vi "PID.vi"(6 "reinitialize? (F)":bool, 7 "output range":cluster{"output high":dbl, "output low":dbl}={"output high"=100.0, "output low"=-100.0} {"output low" format="%.2f"; "output high" format="%.2f"}, 8 "dt (s)":dbl=-1.0 format="%.3f", 9 "PID gains":T1={"proportional gain (Kc)"=1.0, "integral time (Ti, min)"=0.01, "derivative time (Td, min)"=0.0} {"derivative time (Td, min)" format="%.3f"; "integral time (Ti, min)" format="%.3f"; "proportional gain (Kc)" format="%.3f"}, 10 "process variable":dbl format="%.2f", 11 "setpoint":dbl format="%.2f") -> (2 "output":dbl format="%.2f")   [LabVIEW 2012]
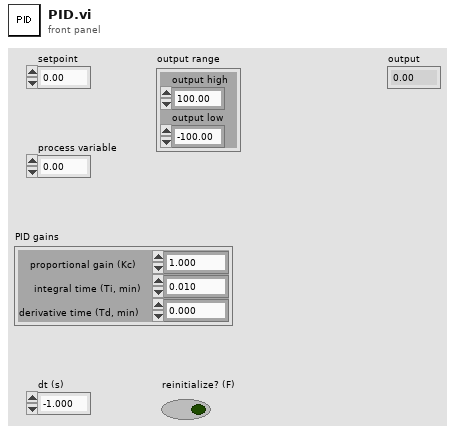
[diagram p1: front panel]
types:
  T1 = cluster{"proportional gain (Kc)":dbl, "integral time (Ti, min)":dbl, "derivative time (Td, min)":dbl}
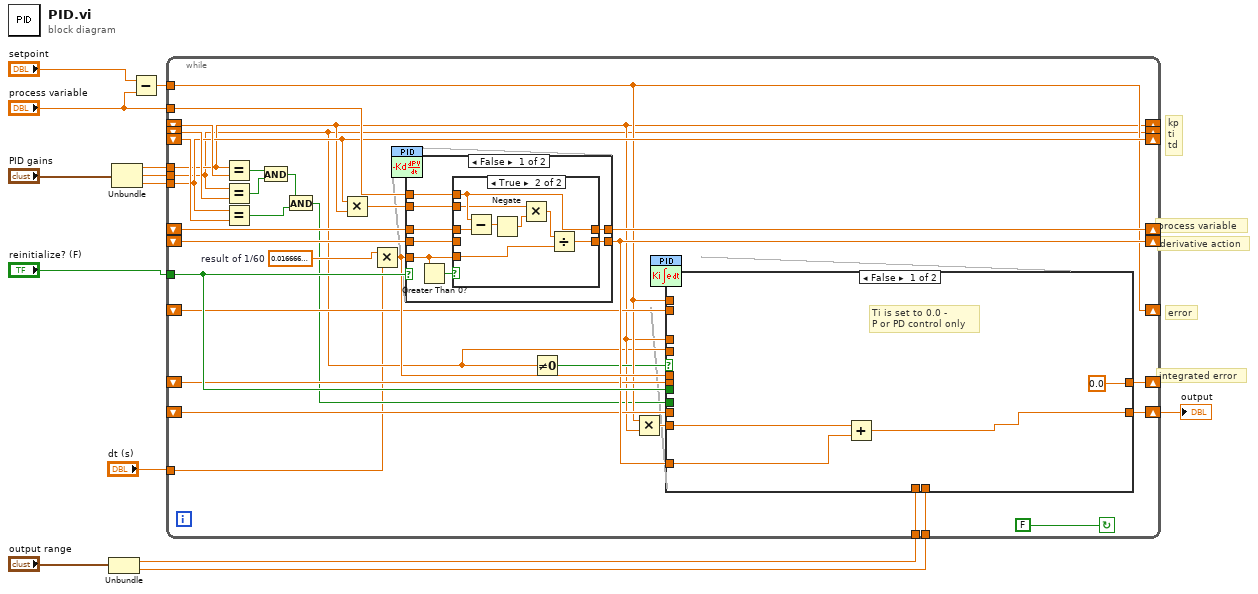
[diagram p0: block diagram]
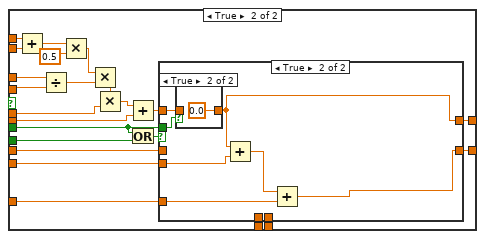
[diagram p2: hidden frame]
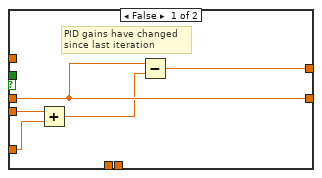
[diagram p3: hidden frame]
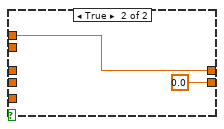
[diagram p6: hidden frame]
diagram:
  # "derivative action"
  # "process variable"
  # "kp\nti\ntd"
  # "error"
  # "integrated error"
  n1 = Unbundle("output range") -> ("output high"=w10:dbl, "output low"=w9:dbl)
  n2 = Unbundle("PID gains") -> ("proportional gain (Kc)"=w13:dbl, "integral time (Ti, min)"=w12:dbl, "derivative time (Td, min)"=w11:dbl)
  n3 = Subtract(x="setpoint", y="process variable") -> (x-y=w2:dbl)
  n4 = while {
    tunnel: "reinitialize? (F)" -> [w45]
    shift-right: [w21] -> _
    shift-left: _ -> [w27]
    shift-right: [w20] -> _
    shift-left: _ -> [w42]
    shift-right: [w25] -> _
    shift-left: _ -> [w43]
    tunnel: w13 -> [w21]
    tunnel: w12 -> [w20]
    tunnel: w11 -> [w25]
    tunnel: "dt (s)" -> [w14]
    tunnel: w10 -> [w41]
    tunnel: w9 -> [w40]
    tunnel: "process variable" -> [w39]
    shift-right: [w38] -> _
    shift-left: _ -> [w37]
    shift-right: [w36] -> _
    shift-left: _ -> [w30]
    shift-right: [w35] -> w6
    shift-left: _ -> [w34]
    shift-right: [w24] -> _
    shift-left: _ -> [w33]
    shift-right: [w32] -> _
    shift-left: _ -> [w31]
    tunnel: w2 -> [w24]
    stop <- FALSE continue-if-true
    w23 = 0.016666666666666666  # result of 1/60
    n5 = Equal?(x=w21, y=w27) -> (x = y?=w19:bool)
    n6 = Equal?(x=w20, y=w42) -> (x = y?=w18:bool)
    n7 = Equal?(x=w25, y=w43) -> (x = y?=w16:bool)
    n8 = And(x=w19, y=w18) -> (x .and. y?=w17:bool)
    n9 = And(x=w17, y=w16) -> (x .and. y?=w15:bool)
    n10 = Multiply(x=w25, y=w21) -> (x*y=w29:dbl)
    n11 = Multiply(x=w23, y=w14) -> (x*y=w44:dbl)
    n12 = case shown="False" w45 {
      tunnel: w37 -> [w94 _]
      tunnel: w29 -> [w91 _]
      tunnel: w39 -> [w93 w106]
      tunnel: [w90 w106] -> w38
      tunnel: [w92 0.0] -> w36
      tunnel: w30 -> [w88 _]
      tunnel: w44 -> [w87 _]
      frame False {
        n13 = Greater Than 0?(x=w87) -> (x > 0?=w89:bool)
        n14 = case shown="True" w89 {
          tunnel: w94 -> [w96 w102]
          tunnel: w87 -> [_ w101]
          tunnel: w93 -> [_ w99]
          tunnel: [w95 w100] -> w92
          tunnel: w91 -> [_ w97]
          tunnel: [w96 w99] -> w90
          tunnel: w88 -> [w95 _]
          frame False {
            # "dt = 0 min"
          }
          frame True {
            n15 = Subtract(x=w99, y=w102) -> (x-y=w104:dbl)
            n16 = Negate(x=w104) -> (-x=w98:dbl)
            n17 = Multiply(x=w97, y=w98) -> (x*y=w103:dbl)
            n18 = Divide(x=w103, y=w101) -> (x/y=w100:dbl)
          }
        }
      }
      frame True {
      }
    }
    n19 = Not Equal To 0?(x=w20) -> (x != 0?=w22:bool)
    n20 = Multiply(x=w24, y=w21) -> (x*y=w28:dbl)
    n21 = case shown="False" w22 {
      tunnel: w24 -> [_ w71]
      tunnel: w33 -> [_ w72]
      tunnel: w31 -> [_ w69]
      tunnel: [0.0 w64] -> w32
      tunnel: w28 -> [w49 w67]
      tunnel: [w46 w63] -> w35
      tunnel: w34 -> [_ w65]
      tunnel: w36 -> [w48 w62]
      tunnel: w45 -> [_ w61]
      tunnel: w15 -> [_ w60]
      tunnel: w44 -> [_ w52]
      tunnel: w41 -> [_ w58]
      tunnel: w40 -> [_ w59]
      tunnel: w21 -> [_ w56]
      tunnel: w20 -> [_ w55]
      frame False {
        # "Ti is set to 0.0 -\nP or PD control only"
        n22 = Add(x=w49, y=w48) -> (x+y=w46:dbl)
      }
      frame True {
        n23 = Add(x=w71, y=w72) -> (x+y=w70:dbl)
        n24 = Divide(x=w56, y=w55) -> (x/y=w53:dbl)
        n25 = Multiply(x=w70, y=0.5) -> (x*y=w54:dbl)
        n26 = Multiply(x=w54, y=w53) -> (x*y=w51:dbl)
        n27 = Multiply(x=w51, y=w52) -> (x*y=w50:dbl)
        n28 = Add(x=w50, y=w69) -> (x+y=w68:dbl)
        n29 = Or(x=w61, y=w60) -> (x .or. y?=w66:bool)
        n30 = case shown="True" w66 {
          tunnel: w68 -> [_ w82]
          tunnel: w67 -> [w75 w81]
          tunnel: w65 -> [w77 _]
          tunnel: w61 -> [_ w83]
          tunnel: [w76 w78] -> w64
          tunnel: [w77 w79] -> w63
          tunnel: w62 -> [w74 w84]
          tunnel: w59 -> [_ _]
          tunnel: w58 -> [_ _]
          frame False {
            # "PID gains have changed\nsince last iteration"
            n31 = Add(x=w75, y=w74) -> (x+y=w73:dbl)
            n32 = Subtract(x=w77, y=w73) -> (x-y=w76:dbl)
          }
          frame True {
            n33 = case shown="True" w83 {
              tunnel: [w85 0.0] -> w78
              tunnel: w82 -> [w85 _]
              frame False {
              }
              frame True {
              }
            }
            n34 = Add(x=w78, y=w81) -> (x+y=w80:dbl)
            n35 = Add(x=w80, y=w84) -> (x+y=w79:dbl)
          }
        }
      }
    }
  }
  "output" <- w6
